vi "EMV T7 Flow Detect 1.vi"(6 "Detect Flow Start?":bool, 8 "error in (no error)":errorcluster, 9 "T7_DELTA_FLOW_THRESHOLD":dbl, 11 "Current T7 Temperatures":dbl[](array[numeric])) -> (0 "error out":errorcluster, 2 "Detection":bool, 3 "Current T7 Temperatures Output":dbl[](array[numeric]))   [LabVIEW 2016]
panel:
  out "slope":dbl
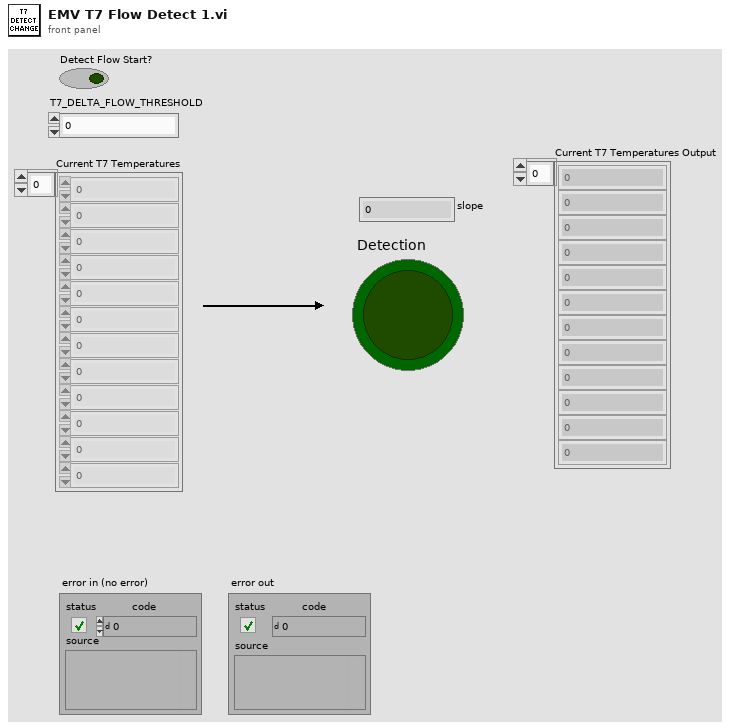
[diagram p1: front panel]
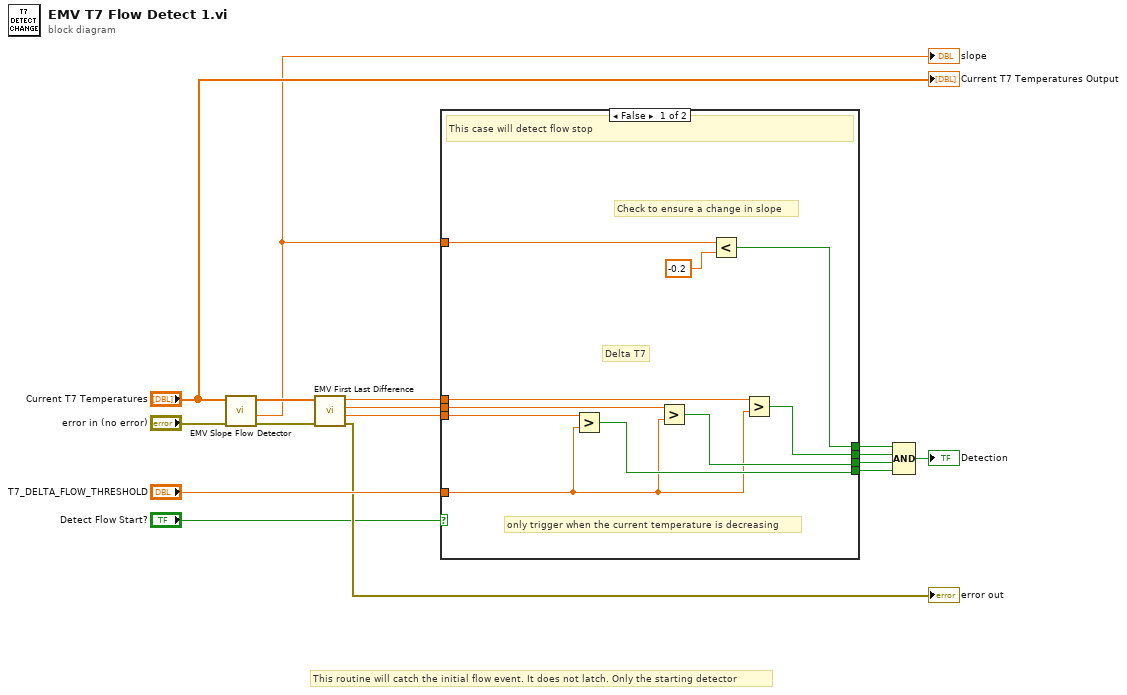
[diagram p0: block diagram]
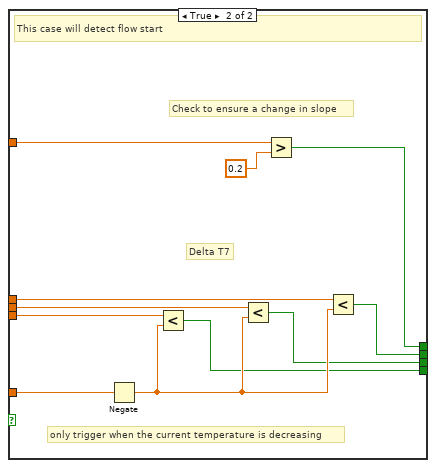
[diagram p2: hidden frame]
diagram:
  # "This routine will catch the initial flow event. It does not latch. Only the starting detector"
  n1 = call "EMV Slope Flow Detector.vi"("error in (no error)"="error in (no error)", "Current T6 Temperatures in"="Current T7 Temperatures") -> ("error out"=w7:errorcluster, "slope"=w4:dbl, "Current T6 Temperatures out"=w6:dbl[])  [unwired: 5 in, 2 out]
  "slope" <- w4
  n2 = call "EMV First Last Difference.vi"("error in (no error)"=w7, "Current T6 Temperatures in"=w6) -> ("error out"=→"error out":errorcluster, "First - Row 8"=w14:dbl, "First - Row 9"=w15:dbl, "First - Row 10"=w16:dbl)  [unwired: 5 in, 1 out]
  n3 = case shown="False" "Detect Flow Start?" {
    tunnel: w16 -> [w22 w37]
    tunnel: w15 -> [w23 w36]
    tunnel: w14 -> [w24 w35]
    tunnel: [w20 w33] -> w13
    tunnel: [w19 w32] -> w12
    tunnel: [w18 w31] -> w11
    tunnel: "T7_DELTA_FLOW_THRESHOLD" -> [w17 w30]
    tunnel: [w21 w29] -> w8
    tunnel: w4 -> [w25 w28]
    frame False {
      # "only trigger when the current temperature is decreasing"
      # "Delta T7"
      # "Check to ensure a change in slope"
      # "This case will detect flow stop"
      n4 = Greater?(x=w24, y=w17) -> (0:w18:bool)
      n5 = Greater?(x=w23, y=w17) -> (0:w19:bool)
      n6 = Less?(x=w25, y=-0.2) -> (x < y?=w21:bool)
      n7 = Greater?(x=w22, y=w17) -> (0:w20:bool)
    }
    frame True {
      # "Check to ensure a change in slope"
      # "only trigger when the current temperature is decreasing"
      # "Delta T7"
      # "This case will detect flow start"
      n8 = Negate(x=w30) -> (-x=w34:dbl)
      n9 = Less?(x=w35, y=w34) -> (x < y?=w31:bool)
      n10 = Less?(x=w36, y=w34) -> (x < y?=w32:bool)
      n11 = Greater?(x=w28, y=0.2) -> (0:w29:bool)
      n12 = Less?(x=w37, y=w34) -> (x < y?=w33:bool)
    }
  }
  n13 = Compound Arithmetic op=AND(w8, w13, w12, w11) -> (→"Detection":bool)
  "Current T7 Temperatures Output" <- "Current T7 Temperatures"
